vi "GetHeuristicCost.vi"(8 "error in (no error)":errorcluster, 10 "Goal NodeReference":refnum<data-value>, 11 "DirectedGraphMapNode in":refnum<class "NI_Robotics_DirectedGraphMapNode.lvclass">) -> (0 "error out":errorcluster, 2 "hueristic cost":dbl, 3 "DirectedGraphMapNode out":refnum<class "NI_Robotics_DirectedGraphMapNode.lvclass">)   [LabVIEW 2017, in "NI_Robotics_DirectedGraphMapNode.lvclass"]
uses:
  <vilib>/robotics/Navigation/shared/MapNode/DirectedGraphMapNode/NI_Robotics_DirectedGraphMapNode.lvclass
  <vilib>/robotics/Navigation/shared/MapNode/AbstractMapNode/NI_Robotics_AbstractMapNode.lvclass
  <vilib>/robotics/Navigation/shared/MapNode/DirectedGraphMapNode/NI_Robotics_DirectedGraphMapNode.lvclass/NI_Robotics_DirectedGraphMapNode.ctl
  <vilib>/robotics/Utilities/NI_Robotics Utilities.lvlib
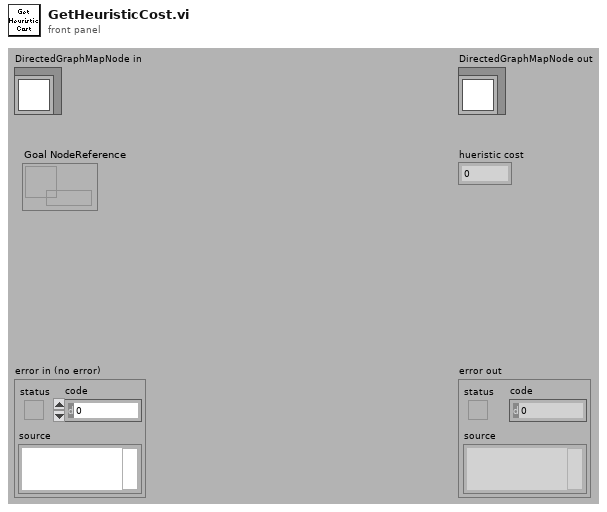
[diagram p1: front panel]
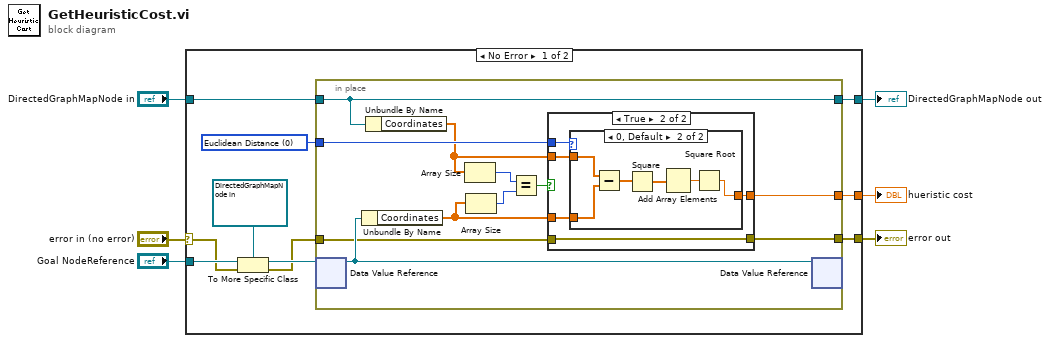
[diagram p0: block diagram]
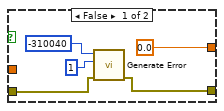
[diagram p2: hidden frame]
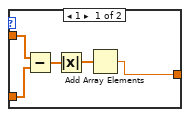
[diagram p3: hidden frame]
diagram:
  n1 = case shown="No Error" "error in (no error)" {
    selector: "error in (no error)" -> [w10 w49]
    tunnel: "Goal NodeReference" -> [w16 _]
    tunnel: [w12 _] -> w5
    tunnel: "DirectedGraphMapNode in" -> [w9 w50]
    tunnel: [w8 w50] -> w3
    tunnel: [w11 w49] -> w2
    frame No Error {
      w7 = u16 0 items=["Euclidean Distance", "Manhattan Distance"] ("heuristic function")
      n2 = To More Specific Class(target class=refnum<data-value> refnum ("data value reference"), reference=w16, error in=w10) -> (specific class reference=w14:refnum<data-value>, error out=w13:errorcluster)
      n3 = in-place {
        in-place-border: w13 -> [w24]
        in-place-border: [w21] -> w12
        in-place-border: [w20] -> w11
        in-place-border: w7 -> [w19]
        in-place-border: w9 -> [w17]
        in-place-border: [w17] -> w8
        n4 = in-place-dvr #1(w14) -> (w27:refnum<class "NI_Robotics_DirectedGraphMapNode.lvclass">)  [unwired: 1 out]
        n5 = Unbundle By Name(w27) -> ("Coordinates"=w23:dbl[])
        n6 = Unbundle By Name(w17) -> ("Coordinates"=w18:dbl[])
        n7 = Array Size(array=w18) -> (size(s)=w26:i32)
        n8 = Array Size(array=w23) -> (size(s)=w25:i32)
        n9 = Equal?(x=w26, y=w25) -> (x = y?=w22:bool)
        n10 = case shown="True" w22 {
          tunnel: w24 -> [w32 w34]
          tunnel: w23 -> [_ w36]
          tunnel: w18 -> [_ w37]
          tunnel: [0.0 ("Hueristic Cost") w35] -> w21
          tunnel: [w28 w34] -> w20
          tunnel: w19 -> [_ w33]
          frame False {
            n11 = call <vilib>:"Generate Error.vi"("error in (no error)"=w32, "chain levels to remove (1)"=1, "code"=-310040) -> ("error out"=w28:errorcluster)  [unwired: 8 in]
          }
          frame True {
            n12 = case shown="0, Default" w33 {
              tunnel: w37 -> [w42 w48]
              tunnel: w36 -> [w41 w47]
              tunnel: [w38 w43] -> w35
              frame 1 {
                n13 = Subtract(x=w42, y=w41) -> (x-y=w40:dbl[])
                n14 = Absolute Value(x=w40) -> (abs(x)=w39:dbl[])
                n15 = Add Array Elements(numeric array=w39) -> (sum=w38:dbl)
              }
              frame 0, Default {
                n16 = Subtract(x=w48, y=w47) -> (x-y=w46:dbl[])
                n17 = Square(x=w46) -> (x^2=w45:dbl[])
                n18 = Add Array Elements(numeric array=w45) -> (sum=w44:dbl)
                n19 = Square Root(x=w44) -> (sqrt(x)=w43:dbl)
              }
            }
          }
        }
        n20 = in-place-dvr #1(w27) -> ()  [unwired: 2 out]
      }
    }
    frame Error {
    }
  }
  "error out" <- w2
  "DirectedGraphMapNode out" <- w3
  "hueristic cost" <- w5
